vi "Read Amplitude (dBm).vi"(8 "error in (no error)":errorcluster, 11 "Microwave in":refnum<class "Microwave.lvclass">) -> (0 "error out":errorcluster, 2 "Amplitude (dBm)":dbl, 3 "Microwave out":refnum<class "Microwave.lvclass">)   [LabVIEW 2017, in "Microwave.lvclass"]
uses:
  Microwave.lvclass
  Microwave.lvclass/Microwave.ctl
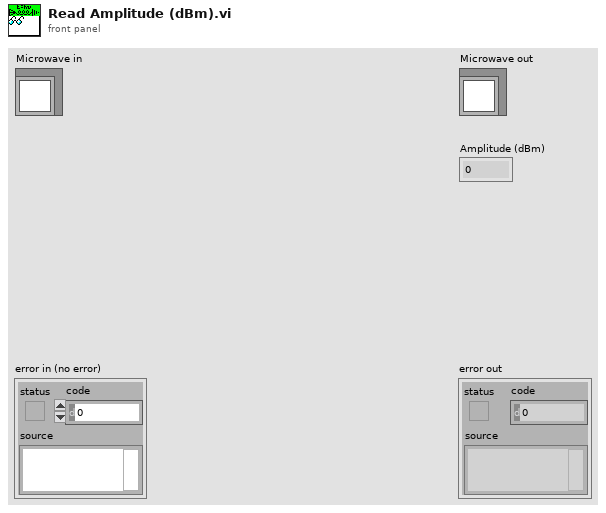
[diagram p1: front panel]
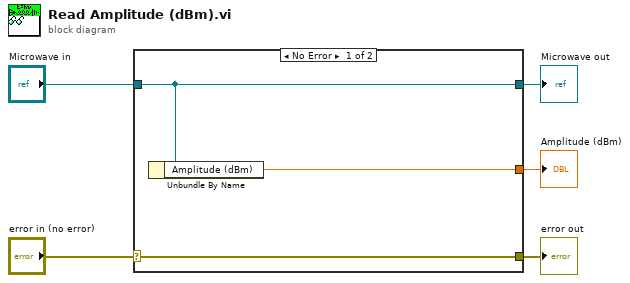
[diagram p0: block diagram]
diagram:
  n1 = case shown="No Error" "error in (no error)" {
    selector: "error in (no error)" -> [w8 w9]
    tunnel: [w8 w9] -> w4
    tunnel: [w7 w10] -> w2
    tunnel: "Microwave in" -> [w7 w10]
    tunnel: [w6 _] -> w1
    frame No Error {
      n2 = Unbundle By Name(w7) -> ("Amplitude (dBm)"=w6:dbl)
    }
    frame Error {
    }
  }
  "error out" <- w4
  "Microwave out" <- w2
  "Amplitude (dBm)" <- w1
